vi "LU_TableMap_Create.vi"(8 "error in":errorcluster, 11 "TableMapping":T1[](array[typedef])) -> (0 "error out":errorcluster, 3 "TableMap":variant)   [LabVIEW 2020, in "ORM_DBC_Kdb.lvlib" / "DBC.lvclass"]
uses:
  DBC.lvclass
  kdb_TableInfo_cluster.ctl
  kdb_TableType_enum.ctl
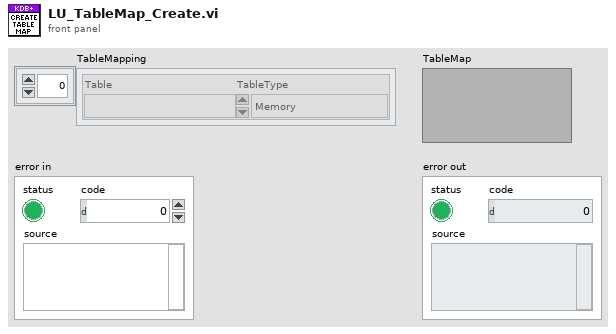
[diagram p1: front panel]
types:
  T1 = typedef "ORM_DBC_Kdb.lvlib/DBC.lvclass/kdb_TableInfo_cluster.ctl" = cluster{"Table":string, "TableType":T2}
  T2 = typedef "ORM_DBC_Kdb.lvlib/DBC.lvclass/kdb_TableType_enum.ctl" = enum16{"Memory", "Disk_Serialized", "Disk_Splayed", "Disk_Partitioned", "Other"}
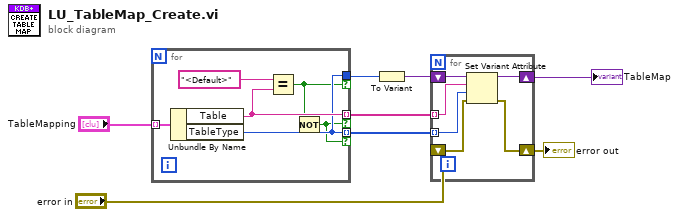
[diagram p0: block diagram]
diagram:
  n1 = for {
    tunnel: "TableMapping" -> [w14] mode=indexing
    tunnel: [w11] -> w4 if=w10
    tunnel: [w12] -> w6 mode=indexing if=w9
    tunnel: [w11] -> w7 mode=indexing if=w9
    n2 = Unbundle By Name(w14) -> ("Table"=w12:string, "TableType"=w11:T2)
    n3 = Equal?(x="<Default>", y=w12) -> (x = y?=w10:bool)
    n4 = Not(x=w10) -> (.not. x?=w9:bool)
  }
  n5 = To Variant(anything=w4) -> (Variant=w5:variant)
  n6 = for {
    tunnel: w6 -> [w19] mode=indexing
    tunnel: w7 -> [w18] mode=indexing
    shift-right: [w17] -> w8
    shift-left: w5 -> [w20]
    shift-right: [w16] -> w2
    shift-left: "error in" -> [w15]
    n7 = Set Variant Attribute(Variant=w20, name=w19, value=w18, error in=w15) -> (Variant out=w17:variant, error out=w16:errorcluster)  [unwired: 1 out]
  }
  "TableMap" <- w8
  "error out" <- w2
